vi "PicoScope6000ExampleBlock_get_waveform&save.vi"() -> ()   [LabVIEW 2016]
uses:
  <vilib>/Analysis/3filter.llb/Filter Passband Type.ctl
  <vilib>/Analysis/2dsp.llb/Real FFT.vi
  <vilib>/Utility/file.llb/Write To Spreadsheet File (I64).vi
  <vilib>/Analysis/3filter.llb/Butterworth Filter (DBL).vi
  ps6000.dll
  <vilib>/Analysis/NI_AALBase.lvlib
  <vilib>/Analysis/NI_AALPro.lvlib
panel:
  in  "Ant / \nPos":bool
  in  "Channel B Settings for trigger":T1={"Enabled"=TRUE, "Coupling"=1, "Range"=6, "Bandwidth"=0, "Analogue Offset"=0.0} {"Bandwidth" items=["Full", "20 MHz"]; "Range" items=["10 mV", "20 mV", "50 mV", "100 mV", "200 mV", "500 mV", "1 V", "2 V", "5 V", "10 V", "20 V", "50 V ", "100 V"]; "Coupling" items=["AC", "DC 1 MOhm", "DC 50 Ohm"]}
  in  "Rapid Block Acquisition Settings":T2={"preTriggerSamples"=0, "postTriggerSamples"=600, "timebase"=5, "Four Channel Device"=FALSE, "Oversample"=1, "Number of Captures"=10000}
  in  "stop":bool
  in  "Monitoring mode":bool=TRUE
  out "Channel A Buffer":i16[][](array[numeric])
  in  "Creat new folder":bool
  out "Ultrasound signal VS Depth":cluster{dbl[], "Channel A Buffer":i16[]}(graph)
  in  "Signal Inverse Switch":bool
  out "Waveform 2":dbl[](graph)
  in  "Waveform low cutoff freq  / Hz":dbl=100.0 format="%0.4f"
  in  "Waveform high cutoff freq / Hz":dbl=10.0 format="%0.2f"
  out "x-y*floor(x/y)":i32
  out "Waveform SF (Hz)":u32
  out "Channel A after H transform":dbl[](graph)
  in  "Start from 2":i32
  in  "length 2":i32=1000
  out "Channel A after filter Zoom-in View":dbl[](graph)
  in  "Folder name":string="test"
  in  "path (use dialog)":path=path "D:/????/2017UCSD??/Ultrasound_Blood_flow_project/Picoscope_Collected_data/20180414"
  in  "STFT Start from":i32
  in  "STFT  length":i32
  out "Channel A after filter Spectrum":dbl[](graph)
  out "millisecond timer value":u32
  out "sampling freq: fs":dbl=78125000.0 format="%0.2f"
  in  "low cutoff freq: fl":dbl=2600000.0 format="%0.4f"
  in  "high cutoff freq: fh":dbl=9000000.0 format="%0.2f"
  out "Channel A after filter":dbl[](graph)
  in  "Acquisition Settings":T3={"preTriggerSamples"=600, "postTriggerSamples"=10000, "timebase"=4, "Down-Sample Mode"=0, "Down Sample Ratio"=1, "Four Channel Device"=FALSE, "Oversample"=1} {"Down Sample Ratio" min=1 step=1; "Down-Sample Mode" items=["None"=0, "Aggregate"=1, "Average"=2, "Decimate"=4, "Distribution"=8]}
  in  "Channel A Settings":T1={"Enabled"=TRUE, "Coupling"=1, "Range"=6, "Bandwidth"=0, "Analogue Offset"=0.0} {"Bandwidth" items=["Full", "20 MHz"]; "Range" items=["10 mV", "20 mV", "50 mV", "100 mV", "200 mV", "500 mV", "1 V", "2 V", "5 V", "10 V", "20 V", "50 V ", "100 V"]; "Coupling" items=["AC", "DC 1 MOhm", "DC 50 Ohm"]}
  in  "Trigger Settings":T4={"Trigger Enabled"=TRUE, "Trigger Source"=enum."Channel A", "Trigger Threshold (16-bit counts)"=31000, "Trigger Direction"=2, "Trigger Delay (samples)"=0, "Auto Trigger Time (ms)"=1000} {"Trigger Direction" items=["Rising"=2, "Falling"=3]}
  out "Channel A":i16[](graph)
  # "Filter Parameters"
  # "FFT data selection"
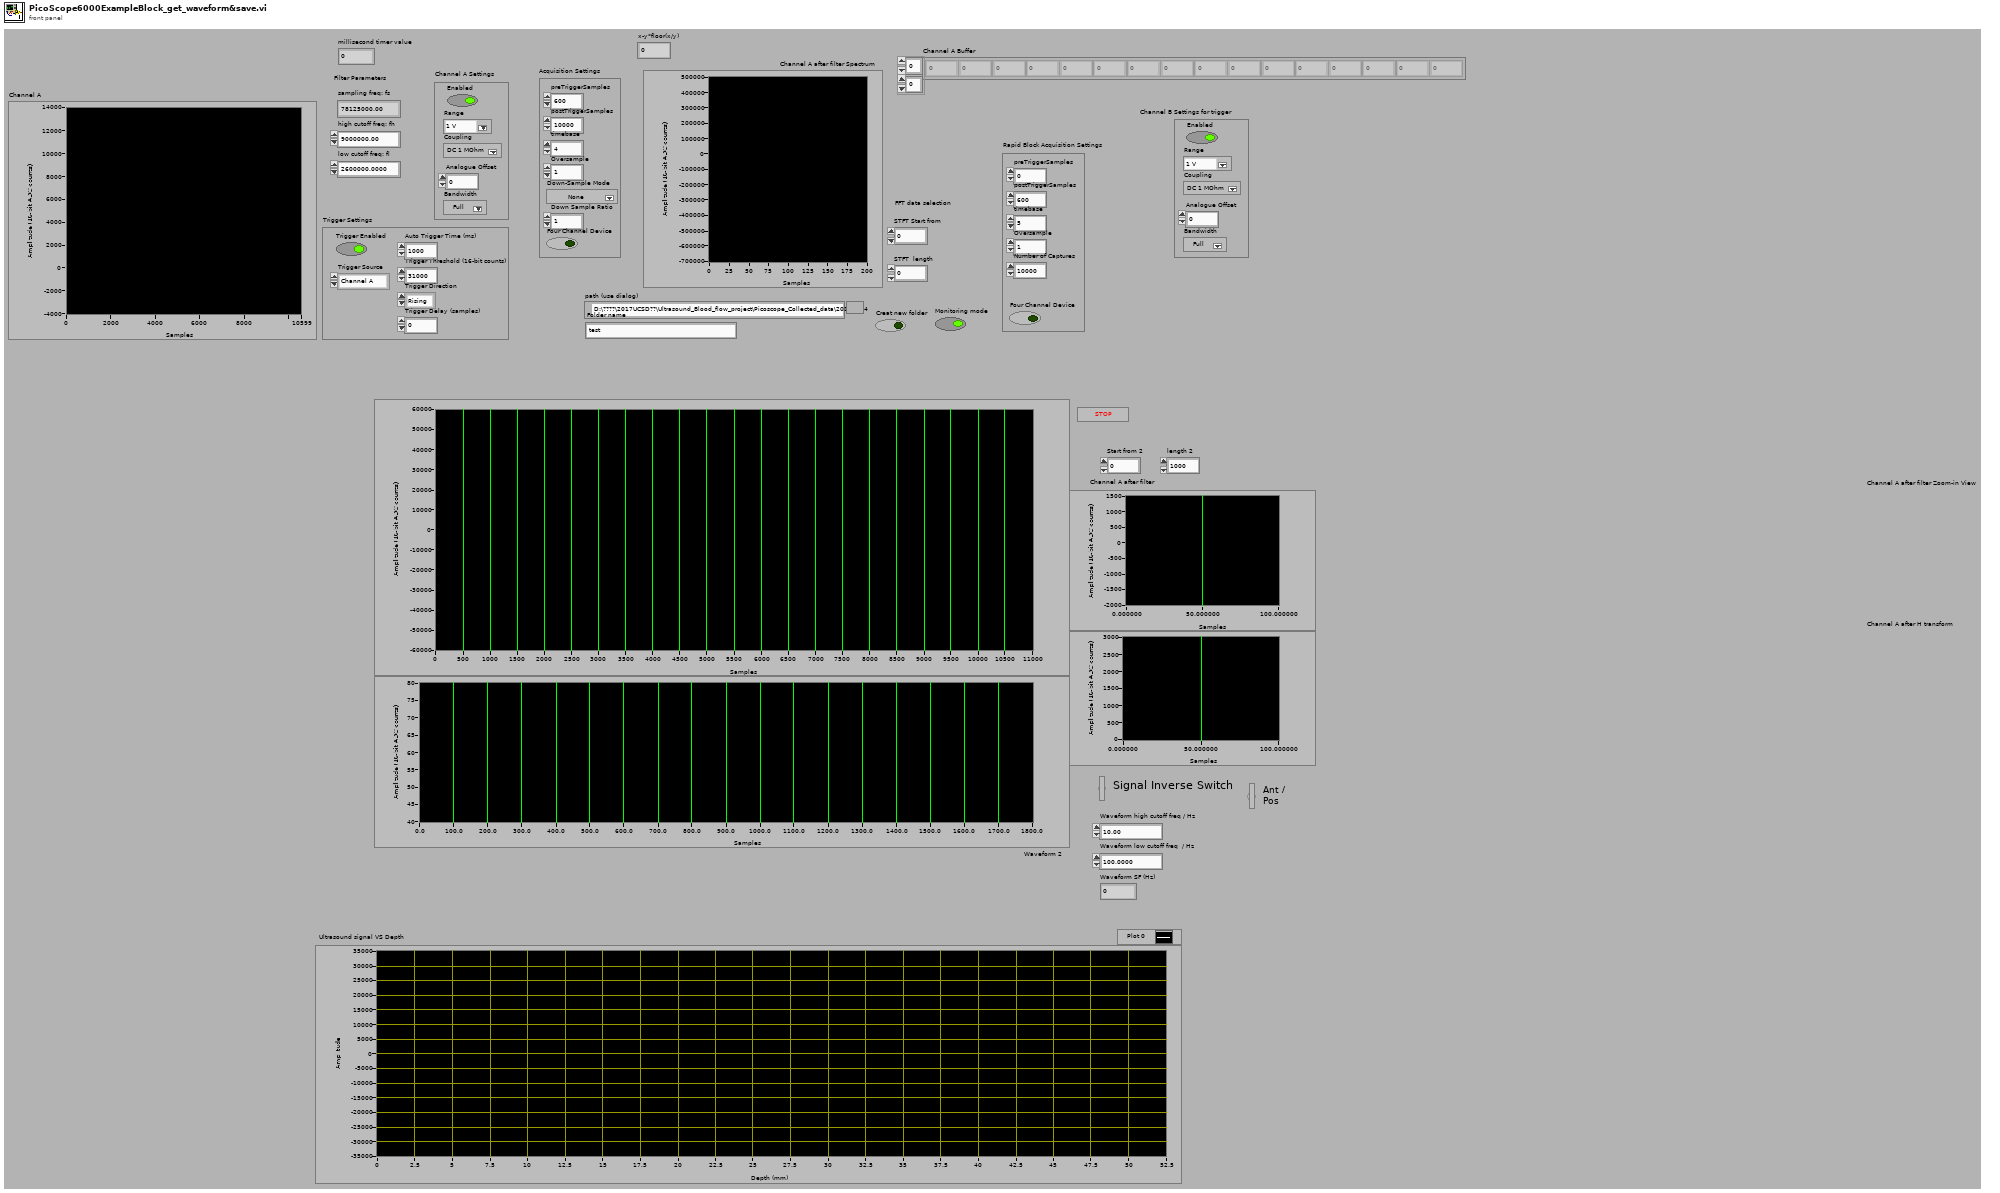
[diagram p1: front panel]
types:
  T1 = cluster{"Enabled":bool, "Coupling":i32, "Range":u16, "Bandwidth":i32, "Analogue Offset":sgl}
  T2 = cluster{"preTriggerSamples":u32, "postTriggerSamples":u32, "timebase":u32, "Four Channel Device":bool, "Oversample":i16, "Number of Captures":u32}
  T3 = cluster{"preTriggerSamples":u32, "postTriggerSamples":u32, "timebase":u32, "Down-Sample Mode":i32, "Down Sample Ratio":u32, "Four Channel Device":bool, "Oversample":i16}
  T4 = cluster{"Trigger Enabled":bool, "Trigger Source":enum16{"Channel A", "Channel B", "Channel C", "Channel D"}, "Trigger Threshold (16-bit counts)":i16, "Trigger Direction":u16, "Trigger Delay (samples)":u32, "Auto Trigger Time (ms)":i16}
  T5 = typedef "NI_AALBase.lvlib/Filter Passband Type.ctl" = enum32{"Lowpass", "Highpass", "Bandpass", "Bandstop"}
  T6 = cluster{"Enabled":bool, "Coupling":i32, "Range":u16, "Analogue Offset":sgl, "Bandwidth":i32}
  T7 = cluster{"Channel D Buffer":i16[], "Channel C Buffer":i16[], "Channel B Buffer":i16[], "Channel A Buffer":i16[]}
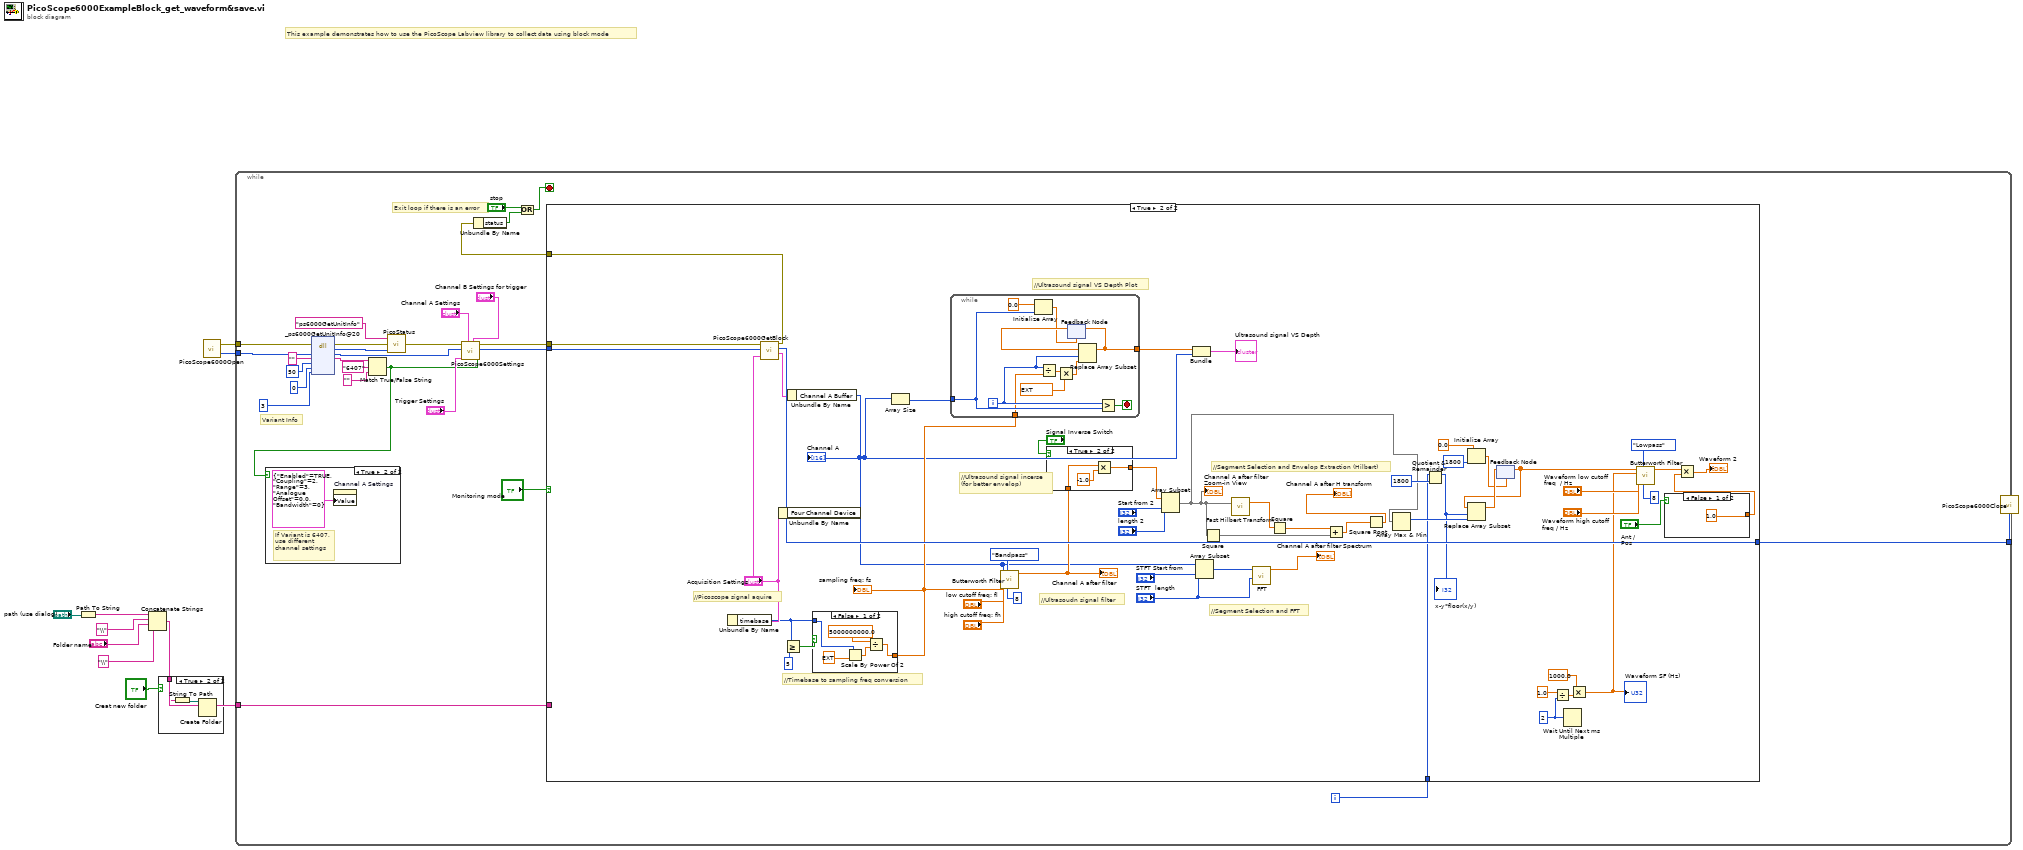
[diagram p0: block diagram]
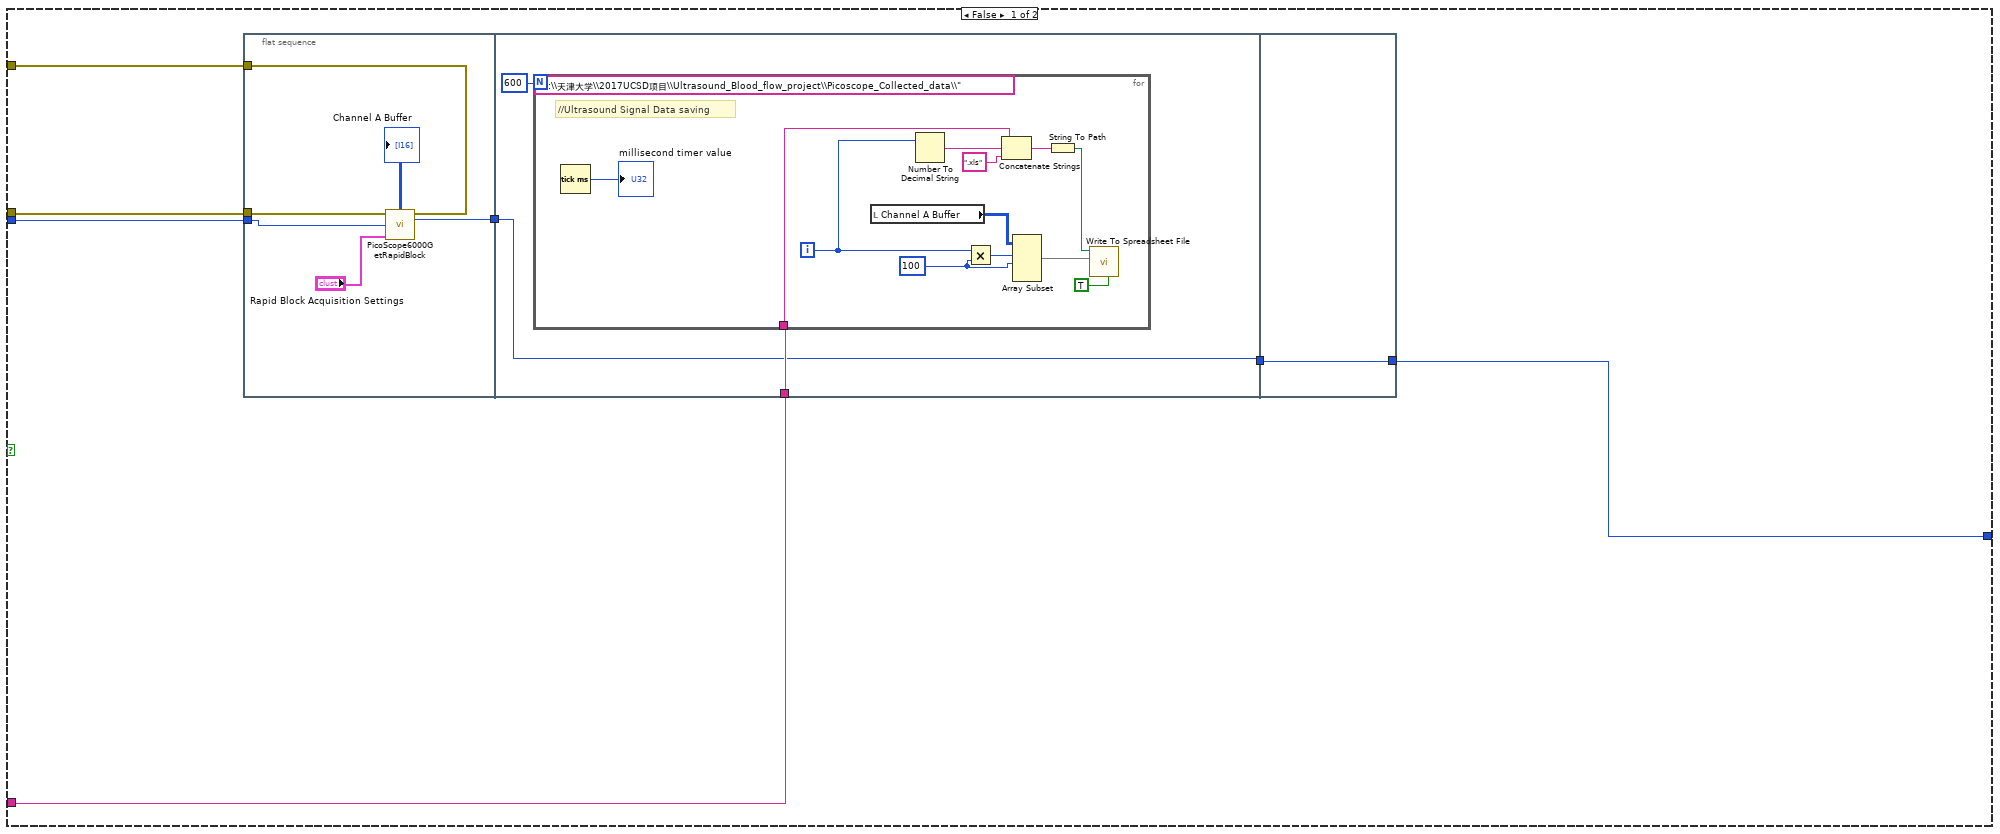
[diagram p3: hidden frame]
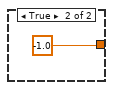
[diagram p4: hidden frame]
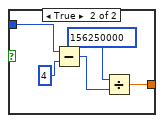
[diagram p6: hidden frame]
diagram:
  # "This example demonstrates how to use the PicoScope Labview library to collect data using block mode"
  n1 = Path To String(path="path (use dialog)") -> (string=w6:string)
  n2 = Concatenate Strings(w6, "\\" ("string"), "Folder name", "\\" ("string")) -> (w1:string)
  n3 = case shown="True" "Creat new folder" {
    tunnel: w1 -> [_ w11]
    frame False {
    }
    frame True {
      n4 = String To Path(string=w11) -> (path=w12:path)
      n5 = Create Folder(path (use dialog)=w12) -> ()  [unwired: 2 in, 3 out]
    }
  }
  n6 = call "PicoScope6000Open.vi"() -> ("error out"=w10:errorcluster, "handle"=w9:i16)  [unwired: 1 in]
  n7 = while {
    tunnel: w9 -> [w36]
    tunnel: [w40] -> w8
    tunnel: w10 -> [w37]
    tunnel: w1 -> [w19]
    i -> [w21]
    stop <- w17 stop-if-true
    # "Exit loop if there is an error"
    # "Variant Info"
    n8 = dll-call lib="C:/SoftwareFiles/LabVIEW Files/Picoscope/picoscope-master/sdk/6000/PS6000.dll" fn="_ps6000GetUnitInfo@20"(error in=w37, "handle"=w36, "string"="", "stringLength"=i16 50, "reqSize"=0, "info"=i16 3) -> (error out=w29:errorcluster, "PICO_STATUS"=w28:i16, "handle"=w26:i16, "string"=w24:string)  [unwired: 5 in, 1 out]
    n9 = Match True/False String(2:"" ("false string"), 3:"6407" ("true string"), 4:w24) -> (0:w18:bool)  [unwired: 1 out]
    n10 = case shown="True" w18 {
      frame False {
      }
      frame True {
        # "If Variant is 6407,\nuse different \nchannel settings"
        n11 = property on="Channel A Settings" class="Clust (strict)"("Value"=T6 {"Enabled"=TRUE, "Coupling"=2, "Range"=3, "Analogue Offset"=0.0, "Bandwidth"=0} ("Channel A Settings")) -> ()  [unwired: 2 in, 2 out]
      }
    }
    n12 = call "PicoStatus.vi"("PICO STATUS"=w28, "error in"=w29, "source"="ps6000GetUnitInfo") -> ("error out"=w27:errorcluster)
    n13 = call "PicoScope6000Settings.vi"("PS6407?"=w18, "Channel B Settings"="Channel B Settings for trigger", "Channel A Settings"="Channel A Settings", "Trigger Settings"="Trigger Settings", "handle in"=w26, "error in"=w27) -> ("handle out"=w23:i16, "error out"=w22:errorcluster)  [unwired: 4 in]
    n14 = case shown="True" "Monitoring mode" {
      tunnel: [w41 w124] -> w40
      tunnel: w23 -> [w46 w78]
      tunnel: w22 -> [w47 w77]
      tunnel: w21 -> [_ w76]
      tunnel: w19 -> [w43 _]
      tunnel: [w45 w75] -> w14
      frame False {
        n15 = flat-sequence {
          tunnel: w47 -> [w51]
          tunnel: w46 -> [w50]
          tunnel: [w49] -> w45
          tunnel: [w48] -> w44
          tunnel: w44 -> [w54]
          tunnel: w43 -> [w55]
          tunnel: [w54] -> w42
          tunnel: w42 -> [w69]
          tunnel: [w69] -> w41
          frame #0 {
            n16 = call "PicoScope6000GetRapidBlock.vi"("error in"=w51, "handle in"=w50, "Rapid Block Acquisition Settings"="Rapid Block Acquisition Settings") -> ("Channel A Buffer"=→"Channel A Buffer":i16[][], "error out"=w49:errorcluster, "handle out"=w48:i16)  [unwired: 7 in, 3 out]
          }
          frame #1 {
            n17 = for {
              N: 600 -> [_]
              tunnel: w55 -> [w61]
              i -> [w57]
              (unwired) "D:\\天津大学\\2017UCSD项目\\Ultrasound_Blood_flow_project\\Picoscope_Collected_data\\" ("字符串")
              w64 = 100 ("x")
              # "//Ultrasound Signal Data saving"
              n18 = Tick Count (ms)() -> (millisecond timer value=→"millisecond timer value":u32)
              n19 = local read "Channel A Buffer"() -> (w59:i16[][])
              n20 = Number To Decimal String(number=w57) -> (decimal integer string=w68:string)  [unwired: 1 in]
              n21 = Multiply(x=w57, y=w64) -> (x*y=w65:i32)
              n22 = Concatenate Strings(w61, w68, ".xls" ("字符串")) -> (w66:string)
              n23 = Array Subset(array=w59, index (row)=w65, length (row)=w64) -> (w58:i16[][])  [unwired: 2 in]
              n24 = String To Path(string=w66) -> (path=w62:path)
              n25 = call-poly <vilib>:"Write To Spreadsheet File.vi"("transpose? (no:F)"=TRUE, "2D data"=w58, "file path (dialog if empty)"=w62) -> ()  [unwired: 5 in, 1 out]
            }
          }
          frame #2 {
          }
        }
      }
      frame True {
        w92 = u32 2 ("millisecond multiple")
        # "//Ultrasoudn signal filter"
        # "//Segment Selection and FFT"
        # "//Segment Selection and Envelop Extraction (Hilbert)"
        # "//Ultrasound signal VS Depth Plot"
        # "//Ultrasound signal incerse\n(for better envelop)"
        # "//Timebase to sampling freq conversion"
        # "//Picoscope signal aquire"
        n26 = Unbundle By Name("Acquisition Settings") -> ("timebase"=w115:u32)
        n27 = call "PicoScope6000GetBlock.vi"("error in"=w77, "handle in"=w78, "Acquisition Settings"="Acquisition Settings") -> ("error out"=w75:errorcluster, "handle out"=w124:i16, "Buffers (Max or non-aggregated)"=w123:T7)  [unwired: 3 in, 2 out]
        n28 = Unbundle By Name("Acquisition Settings") -> ()  [unwired: 1 out]
        n29 = Greater Or Equal?(x=w115, y=u32 5) -> (x >= y?=w116:bool)
        n30 = Unbundle By Name(w123) -> ("Channel A Buffer"=w82:i16[])
        "Channel A" <- w82
        n31 = case shown="False" w116 {
          tunnel: w115 -> [w142 w151]
          tunnel: [w143 w147] -> w84
          frame False {
            n32 = Scale By Power Of 2(n=w142, x=ext 1.0) -> (x*2^n=w144:ext)
            n33 = Divide(x=5000000000.0, y=w144) -> (x/y=w143:ext)
          }
          frame True {
            n34 = Subtract(x=w151, y=u32 4) -> (x-y=w148:u32)
            n35 = Divide(x=u32 156250000 ("y"), y=w148) -> (x/y=w147:dbl)
          }
        }
        "sampling freq: fs" <- w84
        n36 = Array Size(array=w82) -> (size(s)=w85:i32)
        n37 = while {
          tunnel: [w134] -> w83
          tunnel: w85 -> [w131]
          tunnel: w84 -> [w130]
          i -> [w133]
          stop <- w132 stop-if-true
          n38 = Initialize Array(0.0 ("element"), w131) -> (w135:dbl[])
          n39 = Divide(x=w133, y=w130) -> (x/y=w129:ext)
          n40 = Multiply(x=w129, y=ext 1500000.0) -> (x*y=w128:ext)
          n41 = feedback #1(w135) -> (w136:dbl[])
          n42 = Replace Array Subset(array=w136, new element=w128, index=w133) -> (w134:dbl[])
          n43 = feedback-in #1(w134) -> ()
          n44 = Greater?(x=w133, y=w131) -> (0:w132:bool)
        }
        n45 = call-poly <vilib>:"Butterworth Filter.vi"("order"=8, "filter type"=Filter_Passband_Type."Bandpass", "low cutoff freq: fl"="low cutoff freq: fl", "high cutoff freq: fh"="high cutoff freq: fh", "sampling freq: fs"=w84, "X"=w82) -> ("Filtered X"=w86:dbl[])  [unwired: 2 in, 1 out]
        "Channel A after filter" <- w86
        n46 = case shown="True" "Signal Inverse Switch" {
          tunnel: w86 -> [w138 w140]
          tunnel: [w138 w139] -> w80
          frame False {
          }
          frame True {
            n47 = Multiply(x=w140, y=-1.0) -> (x*y=w139:dbl[])
          }
        }
        n48 = Array Subset(array=w80, index="Start from 2", length="length 2") -> (w70:dbl[])
        "Channel A after filter Zoom-in View" <- w70
        n49 = Bundle(w83, "Channel A Buffer"=w82) -> (→"Ultrasound signal VS Depth":cluster{dbl[], "Channel A Buffer":i16[]})  [unwired: 1 in]
        n50 = Array Subset(array=w82, index="STFT Start from", length="STFT  length") -> (w111:i16[])
        n51 = Square(x=w70) -> (x^2=w106:dbl[])
        n52 = call <vilib>:"Fast Hilbert Transform.vi"("X"=w70) -> ("Hilbert{X}"=w108:dbl[])  [unwired: 1 out]
        n53 = call-poly <vilib>:"FFT.vi"("FFT size"="STFT  length", "X"=w111) -> ("FFT {X}"=→"Channel A after filter Spectrum":cdb[])  [unwired: 8 in, 1 out]
        n54 = Square(x=w108) -> (x^2=w107:dbl[])
        n55 = Add(x=w107, y=w106) -> (x+y=w105:dbl[])
        n56 = Square Root(x=w105) -> (sqrt(x)=→"Channel A after H transform":dbl[])
        n57 = Array Max & Min(array=w70) -> (max index (indices)=w103:i32)  [unwired: 3 out]
        n58 = Quotient & Remainder(x=w76, y=1800) -> (x-y*floor(x/y)=w102:i32)  [unwired: 1 out]
        "x-y*floor(x/y)" <- w102
        n59 = Initialize Array(0.0 ("element"), 1800 ("dimension size")) -> (w98:dbl[])
        n60 = feedback #2(w98) -> (w88:dbl[])
        n61 = Replace Array Subset(array=w88, new element=w103, index=w102) -> (w101:dbl[])
        n62 = feedback-in #2(w101) -> ()
        n63 = Divide(x=1.0, y=w92) -> (x/y=w91:dbl)
        n64 = Wait Until Next ms Multiple(millisecond multiple=w92) -> ()  [unwired: 1 out]
        n65 = Multiply(x=1000.0, y=w91) -> (x*y=w89:dbl)
        "Waveform SF (Hz)" <- w89
        n66 = call-poly <vilib>:"Butterworth Filter.vi"("order"=8, "filter type"=Filter_Passband_Type."Lowpass", "low cutoff freq: fl"="Waveform low cutoff freq  / Hz", "high cutoff freq: fh"="Waveform high cutoff freq / Hz", "sampling freq: fs"=w89, "X"=w88) -> ("Filtered X"=w74:dbl[])  [unwired: 2 in, 1 out]
        n67 = case shown="False" "Ant / \nPos" {
          tunnel: [1.0 ("y") -1.0 ("y")] -> w71
          frame False {
          }
          frame True {
          }
        }
        n68 = Multiply(x=w74, y=w71) -> (x*y=→"Waveform 2":dbl[])
      }
    }
    n69 = Unbundle By Name(w14) -> ("status"=w15:bool)
    n70 = Or(x="stop", y=w15) -> (x .or. y?=w17:bool)
  }
  n71 = call "PicoScope6000Close.vi"("handle"=w8) -> ()
